vi "Write Control Description.vi"(8 "error in (no error)":errorcluster, 9 "variant":variant, 11 "VI Description in":string) -> (0 "error out":errorcluster, 3 "VI Description out":string)   [LabVIEW 2019, in "JSON-Schema.lvlib"]
uses:
  JSON-Schema.lvlib
  <vilib>/Utility/Data Type/NI_Data Type.lvlib
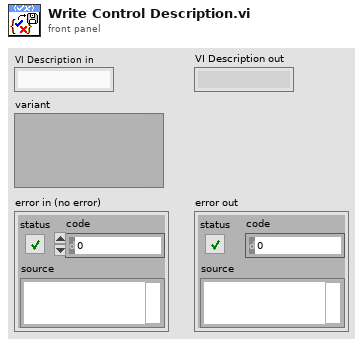
[diagram p1: front panel]
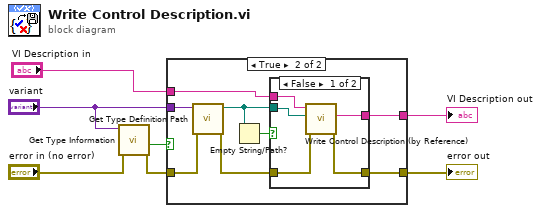
[diagram p0: block diagram]
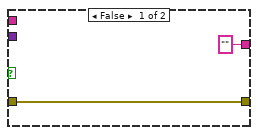
[diagram p2: hidden frame]
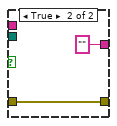
[diagram p3: hidden frame]
diagram:
  n1 = call <vilib>:"Get Type Information.vi"("error in (no error)"="error in (no error)", "variant"="variant") -> ("error out"=w3:errorcluster, "type definition"=w2:bool)  [unwired: 5 in, 3 out]
  n2 = case shown="True" w2 {
    tunnel: [w8 w13] -> w7
    tunnel: ["" ("VI Description") w17] -> w6
    tunnel: "variant" -> [_ w15]
    tunnel: w3 -> [w8 w14]
    tunnel: "VI Description in" -> [_ w10]
    frame False {
    }
    frame True {
      n3 = call <vilib>:"Get Type Definition Path.vi"("error in (no error)"=w14, "variant"=w15) -> ("error out"=w16:errorcluster, "type definition path"=w11:path)  [unwired: 8 in]
      n4 = Empty String/Path?(string/path=w11) -> (empty?=w12:bool)
      n5 = case shown="False" w12 {
        tunnel: [w21 "" ("VI Description")] -> w17
        tunnel: w16 -> [w22 w24]
        tunnel: w11 -> [w19 _]
        tunnel: [w20 w24] -> w13
        tunnel: w10 -> [w18 _]
        frame False {
          n6 = call "Write Control Description (by Reference).vi"("error in (no error)"=w22, "ctl path"=w19, "VI Description in"=w18) -> ("error out"=w20:errorcluster, "VI Description out"=w21:string)  [unwired: 7 in]
        }
        frame True {
        }
      }
    }
  }
  "error out" <- w7
  "VI Description out" <- w6
